vi "updateArrays_pos_names_status.vi"(10 "#ofChannels":i32=7, 11 "name/data 2":string[][](array[string])) -> (0 "Mode":T1[](array[typedef]), 1 "Status":u32[](array[colorbox]), 2 "Names":string[](array[string]), 3 "pos":T2[](array[typedef]))   [LabVIEW 2013]
uses:
  Device Drivers/FilterWheels/posTypDef.ctl
  Device Drivers/FilterWheels/ModeTypDEf.ctl
panel:
  out "Numeric 2":i32
  out "Numeric":i32
  out "subarray":string[](array[string])
  out "Array 3":string[][](array[string])
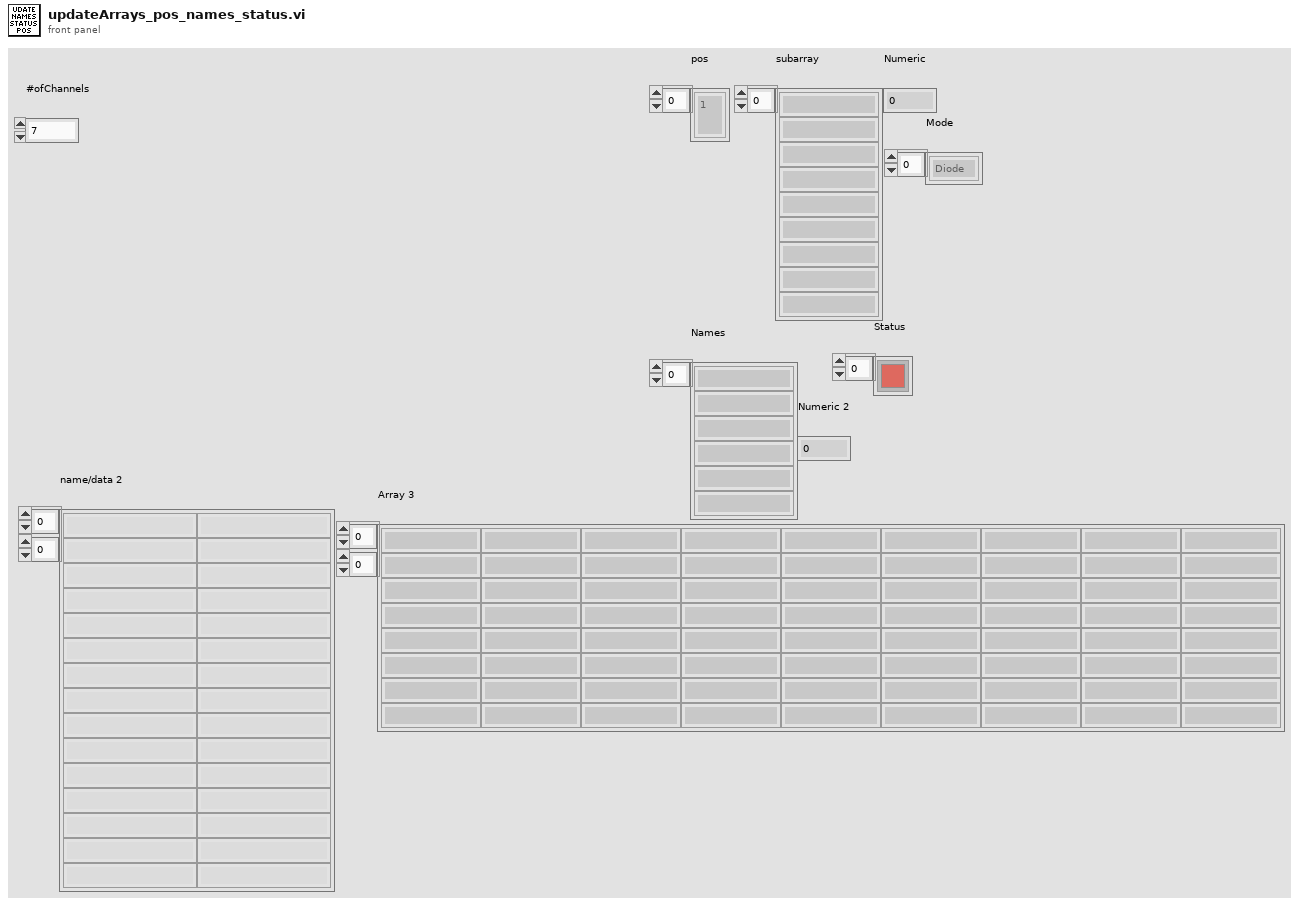
[diagram p1: front panel]
types:
  T1 = typedef "ModeTypDEf.ctl" = enum16{"Diode", "Low Power", "High Power", "undefined"}
  T2 = typedef "posTypDef.ctl" = enum16{"1", "2", "3", "4", "5", "6"}
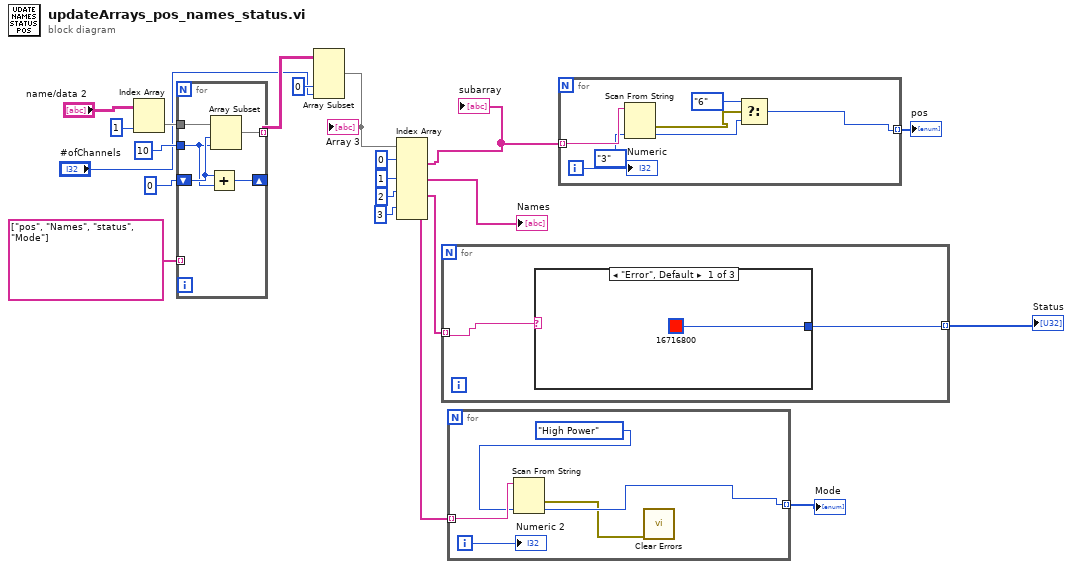
[diagram p0: block diagram]
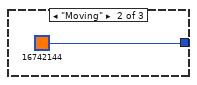
[diagram p2: hidden frame]
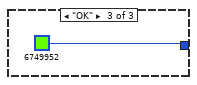
[diagram p3: hidden frame]
diagram:
  n1 = Index Array(array="name/data 2", index (col)=1 ("disabled index (col)")) -> (element=w19:string[])  [unwired: 1 in]
  n2 = for {
    tunnel: string[] ["pos", "Names", "status", "Mode"] -> [_] mode=indexing
    tunnel: w19 -> [w23]
    shift-right: [w24] -> _
    shift-left: 0 ("offset past match") -> [w26]
    tunnel: 10 ("#ofChannels") -> [w25]
    tunnel: [w22] -> w4 mode=indexing
    n3 = Add(x=w26, y=w25) -> (x+y=w24:i32)
    n4 = Array Subset(array=w23, index=w26, length=w25) -> (w22:string[])
  }
  n5 = Array Subset(array=w4, index (col)=0 ("index"), length (col)="#ofChannels") -> (w1:string[][])  [unwired: 2 in]
  "Array 3" <- w1
  n6 = Index Array(array=w1, index (row) #1=0 ("index (row)"), index (row) #2=1 ("index (row)"), index (row) #3=2 ("index (row)"), index (row) #4=3 ("index (row)")) -> (element #1=w11:string[], element #2=→"Names":string[], element #3=w12:string[], element #4=w8:string[])  [unwired: 4 in]
  "subarray" <- w11
  n7 = for {
    tunnel: w12 -> [w28] mode=indexing
    tunnel: [w27] -> w6 mode=indexing
    n8 = case shown="\"Error\", Default" w28 {
      tunnel: [u32 16716800 u32 16742144 u32 6749952] -> w27
      frame "Error", Default {
      }
      frame "Moving" {
      }
      frame "OK" {
      }
    }
  }
  "Status" <- w6
  n9 = for {
    tunnel: w8 -> [w36] mode=indexing
    tunnel: [w33] -> w7 mode=indexing
    i -> [w35]
    n10 = Scan From String(input string=w36, default 1=ModeTypDEf."High Power" ("Mode")) -> (error out=w32:errorcluster, output 1=w33:T1)  [unwired: 3 in, 2 out]
    n11 = call <vilib>:"Clear Errors.vi"("error in (no error)"=w32) -> ()  [unwired: 6 in, 1 out]
    "Numeric 2" <- w35
  }
  "Mode" <- w7
  n12 = for {
    tunnel: w11 -> [w43] mode=indexing
    tunnel: [w38] -> w10 mode=indexing
    i -> [w41]
    n13 = Scan From String(input string=w43, default 1=posTypDef."3" ("Channel1")) -> (error out=w40:errorcluster, output 1=w39:T2)  [unwired: 3 in, 2 out]
    n14 = Select(t=posTypDef."6", s=w40, f=w39) -> (s? t:f=w38:T2)
    "Numeric" <- w41
  }
  "pos" <- w10
